vi "Write filter.vi"(8 "error in (no error)":errorcluster, 10 "filter":bool, 11 "CRDS in":refnum<class "CRDS Data.lvclass">) -> (0 "error out":errorcluster, 3 "CRDS out":refnum<class "CRDS Data.lvclass">)   [LabVIEW 2014, in "CRDS Lib.lvlib" / "CRDS Data.lvclass"]
uses:
  CRDS Data.lvclass
  CRDS Data.lvclass/CRDS Data.ctl
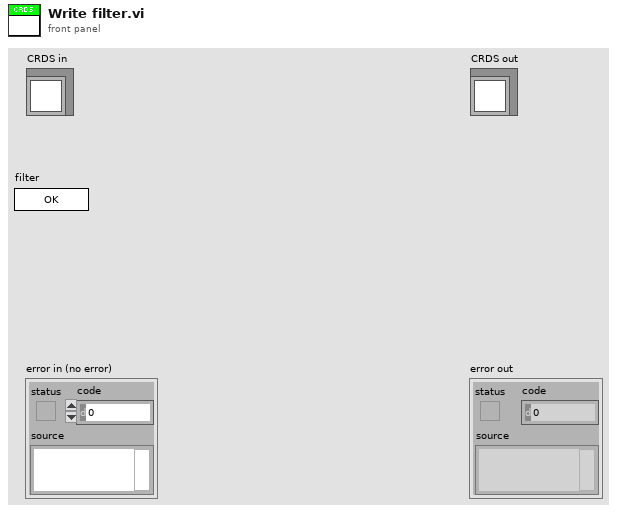
[diagram p1: front panel]
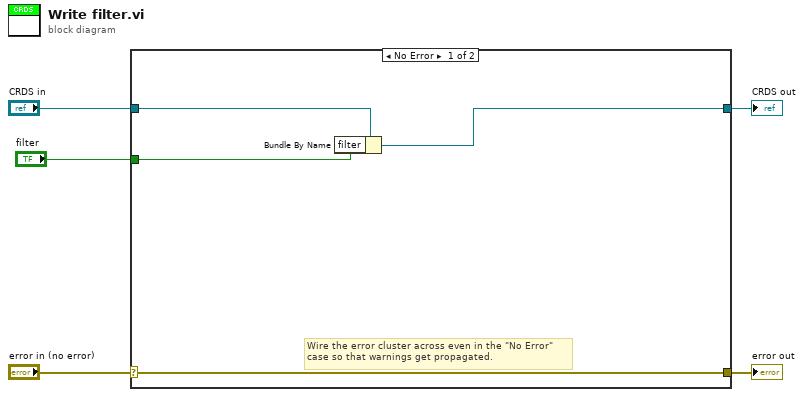
[diagram p0: block diagram]
diagram:
  n1 = case shown="No Error" "error in (no error)" {
    selector: "error in (no error)" -> [w9 w11]
    tunnel: [w9 w11] -> w4
    tunnel: [w6 w10] -> w2
    tunnel: "CRDS in" -> [w7 w10]
    tunnel: "filter" -> [w8 _]
    frame No Error {
      # "Wire the error cluster across even in the \"No Error\"\ncase so that warnings get propagated."
      n2 = Bundle By Name(cluster=w7, "filter"=w8) -> (w6:refnum<class "CRDS Data.lvclass">)
    }
    frame Error {
    }
  }
  "error out" <- w4
  "CRDS out" <- w2
